vi "Read Name.vi"(8 "Error In":errorcluster, 11 "Known Host In":refnum<class "KnownHost.lvclass">) -> (0 "Error Out":errorcluster, 2 "Name":string, 3 "Known Host Out":refnum<class "KnownHost.lvclass">)   [LabVIEW 2017, in "Toolkit.lvlib" / "KnownHost.lvclass"]
uses:
  KnownHost.lvclass
  KnownHost.lvclass/KnownHost.ctl
  Toolkit.lvlib
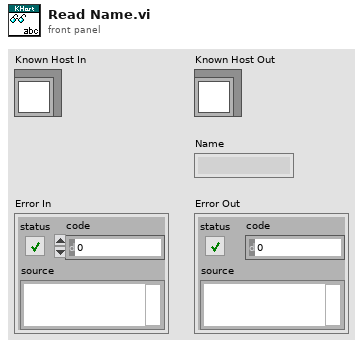
[diagram p1: front panel]
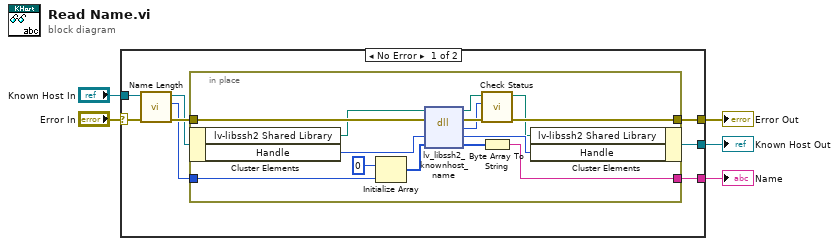
[diagram p0: block diagram]
diagram:
  n1 = case shown="No Error" "Error In" {
    selector: "Error In" -> [w11 w29]
    tunnel: [w13 w29] -> w4
    tunnel: "Known Host In" -> [w9 w28]
    tunnel: [w12 w28] -> w2
    tunnel: [w6 _] -> w1
    frame No Error {
      n2 = call "Name Length.vi"("Error In"=w11, "Known Host In"=w9) -> ("Error Out"=w10:errorcluster, "Length"=w7:u64, "Known Host Out"=w8:refnum<class "KnownHost.lvclass">)  [unwired: 7 in]
      n3 = in-place {
        in-place-border: w10 -> [w27]
        in-place-border: [w22] -> w13
        in-place-border: w7 -> [w17]
        in-place-border: [w14] -> w6
        n4 = in-place-cluster #1(w8) -> ("lv-libssh2 Shared Library"=w26:path, "Handle"=w25:u64)
        n5 = Initialize Array(u8 0, w17) -> (w16:u8[])
        n6 = dll-call lib="lv-libssh2.*" fn="lv_libssh2_knownhost_name"(path in=w26, error in=w27, "handle"=w25, "buffer"=w16) -> (path out=w21:path, error out=w23:errorcluster, "status"=w19:i32, "handle"=w24:u64, "buffer"=w15:u8[])  [unwired: 1 in]
        n7 = call "Check Status.vi"("Error In"=w23, "Status"=w19, "lv-libssh2 Shared Library In"=w21) -> ("Error Out"=w22:errorcluster, "lv-libssh2 Shared Library Out"=w20:path)  [unwired: 7 in]
        n8 = Byte Array To String(unsigned byte array=w15) -> (string=w14:string)
        n9 = in-place-cluster #1("lv-libssh2 Shared Library"=w20, "Handle"=w24) -> (w12:refnum<class "KnownHost.lvclass">)
      }
    }
    frame Error {
    }
  }
  "Error Out" <- w4
  "Known Host Out" <- w2
  "Name" <- w1
